vi "Aspect Ratio Square.vi"(8 "Bottom Left":dbl, 9 "Top Left":dbl, 10 "Bottom Right":dbl, 11 "Top Right":dbl) -> (3 "Score":dbl)   [LabVIEW 2020]
doc: "This VI compares the calculated diameter and convex hull area to compare this shape to a half-hexagon."
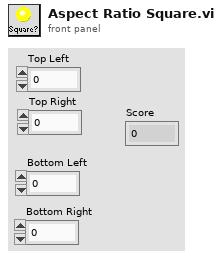
[diagram p1: front panel]
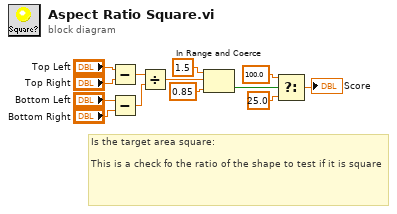
[diagram p0: block diagram]
diagram:
  # "Is the target area square:\n\nThis is a check fo the ratio of the shape to test if it is square"
  n1 = Subtract(x="Top Left", y="Top Right") -> (x-y=w10:dbl)
  n2 = Subtract(x="Bottom Left", y="Bottom Right") -> (x-y=w11:dbl)
  n3 = Divide(x=w10, y=w11) -> (x/y=w7:dbl)
  n4 = In Range and Coerce(upper limit=1.5, x=w7, lower limit=0.85) -> (In Range?=w4:bool)  [unwired: 1 out]
  n5 = Select(t=100.0, s=w4, f=25.0) -> (s? t:f=→"Score":dbl)
